vi "JKI Get Web Browser Path__jki_lib_communication -- VI Tester.vi"(4 "error in (no error)":errorcluster) -> (0 "error out":errorcluster, 3 "browser command":string)   [LabVIEW 2011]
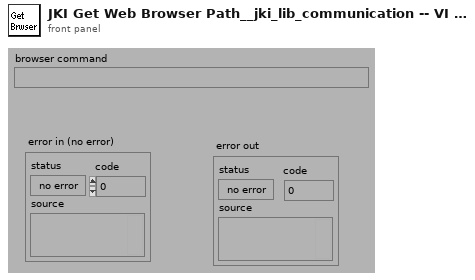
[diagram p1: front panel]
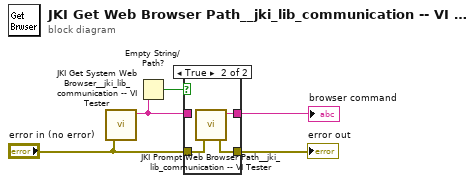
[diagram p0: block diagram]
diagram:
  n1 = call "JKI Get System Web Browser__jki_lib_communication -- VI Tester.vi"("error in (no error)"="error in (no error)") -> ("browser command"=w1:string)  [unwired: 5 in, 1 out]
  n2 = Empty String/Path?(string/path=w1) -> (empty?=w4:bool)
  n3 = case shown="True" w4 {
    tunnel: "error in (no error)" -> [w7 w10]
    tunnel: [w7 w9] -> w3
    tunnel: [w6 w8] -> w2
    tunnel: w1 -> [w6 _]
    frame False {
    }
    frame True {
      n4 = call "JKI Prompt Web Browser Path__jki_lib_communication -- VI Tester.vi"("error in (no error)"=w10) -> ("error out"=w9:errorcluster, "browser path"=w8:string)  [unwired: 5 in]
    }
  }
  "browser command" <- w2
  "error out" <- w3
